vi "N5224B_Meas (SubVI).vi"(8 "error in (no error)":errorcluster, 9 "Sample Count (401)":u32=11, 11 "VISA Refnum in":refnum<visa-resource-name>) -> (0 "Error Out":errorcluster, 2 "Phase":dbl[](array[numeric]), 3 "Gain":dbl[](array[numeric]))   [LabVIEW 2020]
uses:
  <instrlib>/Agilent PNA Series/Agilent PNA Series.lvlib
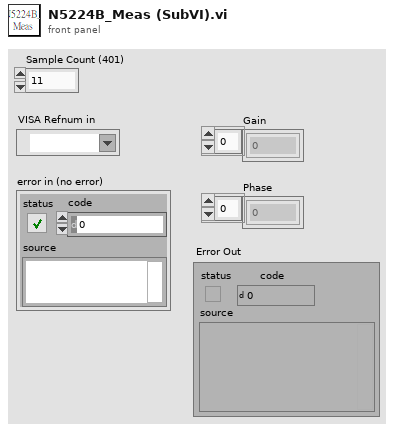
[diagram p1: front panel]
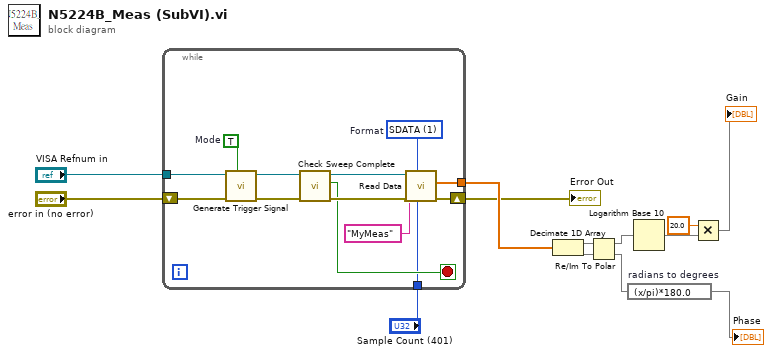
[diagram p0: block diagram]
diagram:
  n1 = while {
    tunnel: "VISA Refnum in" -> [w23]
    tunnel: [w21] -> w3
    shift-right: [w20] -> w2
    shift-left: "error in (no error)" -> [w22]
    tunnel: "Sample Count (401)" -> [w14]
    stop <- w15 stop-if-true
    w16 = TRUE  # Mode
    w26 = u16 1 items=["FDATA", "SDATA", "FMEM", "SMEM", "SDIV"]  # Format
    n2 = call <instrlib>:"Generate Trigger Signal.vi"("Mode (T: Initiate)"=w16, "Error In (no error)"=w22, "VISA Resource Name"=w23) -> ("Error Out"=w17:errorcluster, "VISA Resource Name Out"=w18:refnum<visa-resource-name>)  [unwired: 7 in]
    n3 = call <instrlib>:"Check Sweep Complete.vi"("Error In (no error)"=w17, "VISA Resource Name"=w18) -> ("Error Out"=w24:errorcluster, "Sweep Complete"=w15:bool, "VISA Resource Name Out"=w25:refnum<visa-resource-name>)  [unwired: 7 in]
    n4 = call <instrlib>:"Read Data.vi"("Sample Count (401)"=w14, "Format  (0: FDATA)"=w26, "Error In (no error)"=w24, "Measurement Name (MY_MEAS)"="MyMeas", "VISA Resource Name"=w25) -> ("Error Out"=w20:errorcluster, "Data"=w21:dbl[])  [unwired: 4 in, 1 out]
  }
  "Error Out" <- w2
  n5 = Decimate 1D Array(w3) -> (w6:dbl[], w7:dbl[])
  n6 = Re/Im To Polar(2:w7, 3:w6) -> (0:w9:dbl[], 1:w8:dbl[])
  n7 = expression code="(x/pi)*180.0" "radians to degrees"(w9) -> (→"Phase":dbl[])
  n8 = Logarithm Base 10(1:w8) -> (0:w10:dbl[])
  n9 = Multiply(x=20.0, y=w10) -> (x*y=→"Gain":dbl[])
